vi "Project Reference By Name.vi"(8 "Error In":errorcluster, 10 "Project Name":string, 11 "App In":refnum<vi>) -> (0 "Error Out":errorcluster, 2 "Project":refnum<vi>, 3 "App Out":refnum<vi>)   [LabVIEW 2018, in "Bookmark Manager.lvlib"]
uses:
  Bookmark Manager.lvlib
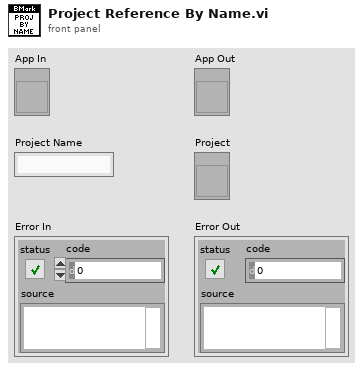
[diagram p1: front panel]
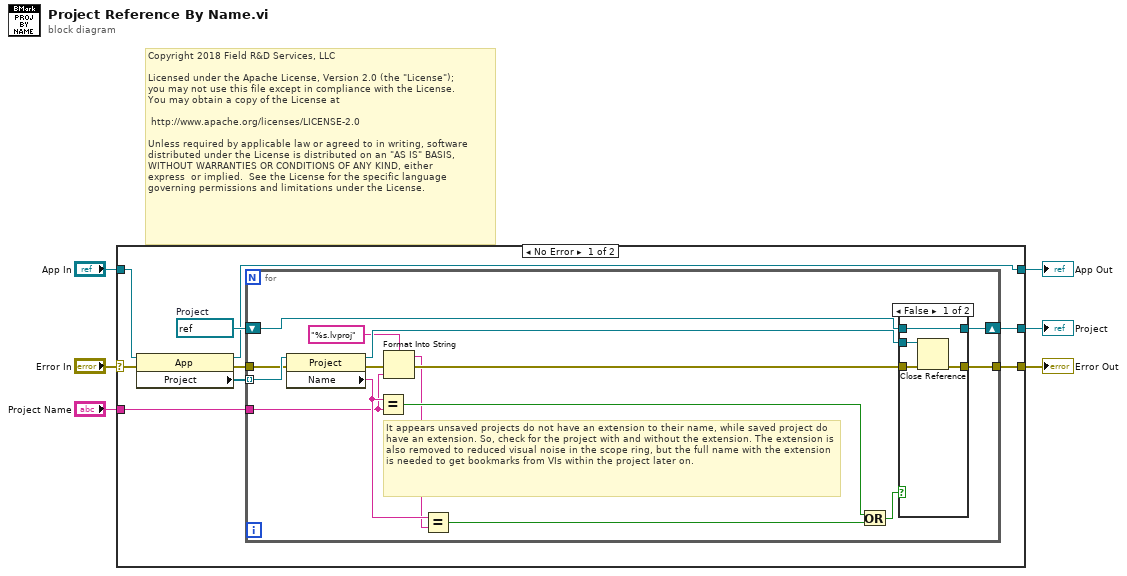
[diagram p0: block diagram]
diagram:
  # "Copyright 2018 Field R&D Services, LLC\n\nLicensed under the Apache License, Version 2.0 (the \"License\");\nyou may not use this file except in compliance with the License.\nYou may obtain a copy of the License at\n\n\thttp://www.apache.org/licenses/LICENSE-2.0\n\nUnless required by applicable law or agreed to in writing, software\ndistributed under the License is distributed on an \"AS IS\" BASIS,\nWITHOUT WARRANTIES OR CONDITIONS OF ANY KIND, either \nexpress  or implied.  See the License for the specific language \ngoverning permissions and limitations under the License."
  n1 = case shown="No Error" "Error In" {
    selector: "Error In" -> [w7 w37]
    tunnel: [w12 w38] -> w6
    tunnel: "App In" -> [w11 w38]
    tunnel: [w10 _] -> w4
    tunnel: "Project Name" -> [w9 _]
    tunnel: [w8 w37] -> w2
    frame No Error {
      w15 = refnum<vi> refnum  # Project
      n2 = property class="App"(reference=w11, error in=w7) -> (reference out=w12:refnum<vi>, error out=w13:errorcluster, "Project"=w14:refnum<vi>[])
      n3 = for {
        tunnel: w13 -> [w29]
        tunnel: w14 -> [w30] mode=indexing
        tunnel: w9 -> [w16]
        tunnel: [w26] -> w8
        shift-right: [w24] -> w10
        shift-left: w15 -> [w25]
        # "It appears unsaved projects do not have an extension to their name, while saved project do have an extension. So, check for the project with and without the extension. The extension is also removed to reduced visual noise in the scope ring, but the full name with the extension is needed to get bookmarks from VIs within the project later on."
        n4 = property class="Project"(reference=w30, error in=w29) -> (reference out=w28:refnum<vi>, error out=w27:errorcluster, "Name"=w21:string)
        n5 = Equal?(x=w21, y=w16) -> (x = y?=w23:bool)
        n6 = Format Into String(format string="%s.lvproj", error in=w27, w16) -> (resulting string=w17:string, error out=w20:errorcluster)  [unwired: 1 in]
        n7 = Equal?(x=w21, y=w17) -> (x = y?=w18:bool)
        n8 = Or(x=w23, y=w18) -> (x .or. y?=w22:bool)
        n9 = case shown="False" w22 {
          tunnel: w28 -> [w33 w36]
          tunnel: w20 -> [w34 w35]
          tunnel: [w32 w35] -> w26
          tunnel: w25 -> [w31 _]
          tunnel: [w31 w36] -> w24
          frame False {
            n10 = Close Reference(reference=w33, error in (no error)=w34) -> (error out=w32:errorcluster)
          }
          frame True {
          }
        }
      }
    }
    frame Error {
    }
  }
  "Project" <- w4
  "Error Out" <- w2
  "App Out" <- w6
